vi "PS Control (OLD).vi"() -> ()   [LabVIEW 2013]
uses:
  <vilib>/rvi/interface/nirviOpenFPGA/nirviOpenFPGA.xnode
  <vilib>/rvi/interface/nirviReadWriteControl/nirviReadWriteControl.xnode
  <vilib>/rvi/interface/Simulation/niFpgaSimulationCallBeginRW.vi
  <vilib>/rvi/errors/niLvFpgaAdjustHostInterfaceError.vi
  <vilib>/addons/control/pid/NI_PID_pid.lvlib
  <vilib>/addons/control/pid/pid.llb/PID (DBL).vi
  <vilib>/ptbypt/NI_PtbyPt.lvlib
  <vilib>/Analysis/3filter.llb/Filter Passband Type.ctl
  <vilib>/Analysis/NI_AALBase.lvlib
  NiFpgaLv.dll
  <vilib>/Utility/error.llb/Error Cluster From Error Code.vi
  <vilib>/NI_Real-Time Target Support.lvlib
  FPGA Bitfiles/TIsbRIO_FPGATarget_pscontroldebug(f_tRBWsiwFJX4.lvbitx
  debug/ps control debug (fpga).vi
  <vilib>/FPGAPlugInAG/sbRIO-9626/niLvFpga_Open_sbRIO-9626.vi
  <vilib>/rvi/interface/common/dynamic/niFpgaDynamicAddResources.vi
panel:
  in  "feedforward":dbl
  out "Total (%)":dbl
  in  "Scale 2":dbl=2.0
  in  "Offset 2":dbl
  out "PS Feedback 2":dbl=1.3965510190723505
  in  "PS Cmd 2":dbl=13.5 format="%.2f"
  in  "PID gains 2":T1={"proportional gain (Kc)"=1.0, "integral time (Ti, min)"=0.01, "derivative time (Td, min)"=0.0} {"derivative time (Td, min)" format="%.3f"; "integral time (Ti, min)" format="%.3f"; "proportional gain (Kc)" format="%.3f"}
  in  "dt (s) 2":dbl=-1.0 format="%.3f"
  in  "output range 2":cluster{"output high":dbl, "output low":dbl}={"output high"=8.0, "output low"=0.0} {"output low" format="%.2f"; "output high" format="%.2f"}
  out "AO1":fxp<+/-,20,5>=0.7481689453125
  out "AI7":fxp<+/-,24,5>=0.5325374603271484
  out "AI6":fxp<+/-,24,5>=0.5325374603271484
  out "AO0":fxp<+/-,20,5>=0.7481689453125
  in  "output range":cluster{"output high":dbl, "output low":dbl}={"output high"=8.0, "output low"=0.0} {"output low" format="%.2f"; "output high" format="%.2f"}
  in  "dt (s)":dbl=-1.0 format="%.3f"
  in  "PID gains":T1={"proportional gain (Kc)"=1.0, "integral time (Ti, min)"=0.01, "derivative time (Td, min)"=0.0} {"derivative time (Td, min)" format="%.3f"; "integral time (Ti, min)" format="%.3f"; "proportional gain (Kc)" format="%.3f"}
  in  "PS Cmd 1":dbl=13.5 format="%.2f"
  out "PS Feedback 1":dbl=1.3965510190723505
  in  "Offset":dbl
  in  "Scale":dbl=2.0
  in  "Loop Timer (uSec)":u32=10000
  # "PS 1"
  # "PS 2"
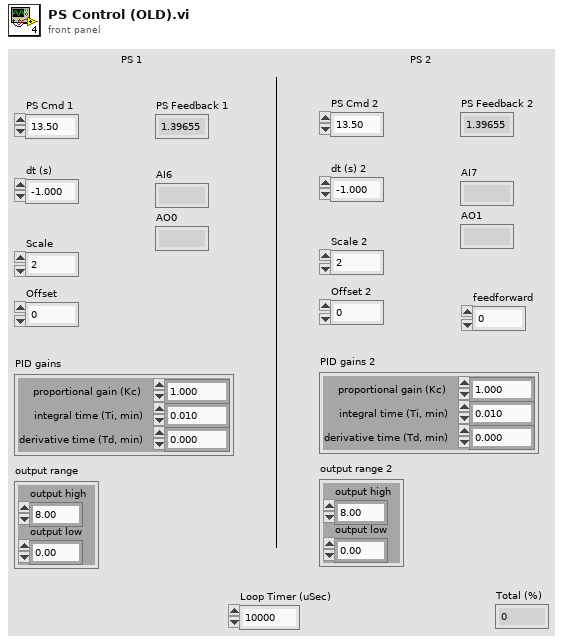
[diagram p1: front panel]
types:
  T1 = cluster{"proportional gain (Kc)":dbl, "integral time (Ti, min)":dbl, "derivative time (Td, min)":dbl}
  T2 = typedef "NI_AALBase.lvlib/Filter Passband Type.ctl" = enum32{"Lowpass", "Highpass", "Bandpass", "Bandstop"}
  T3 = typedef "NI_Real-Time Target Support.lvlib/RT CPU Load.ctl" = cluster{"Total (%)":dbl, "Time Critical (%)":dbl, "Timed Structures (%)":dbl, "High (%)":dbl, "Above Normal (%)":dbl, "Normal (%)":dbl, "Background (%)":dbl, "Idle (%)":dbl, "ISR (%)":dbl}
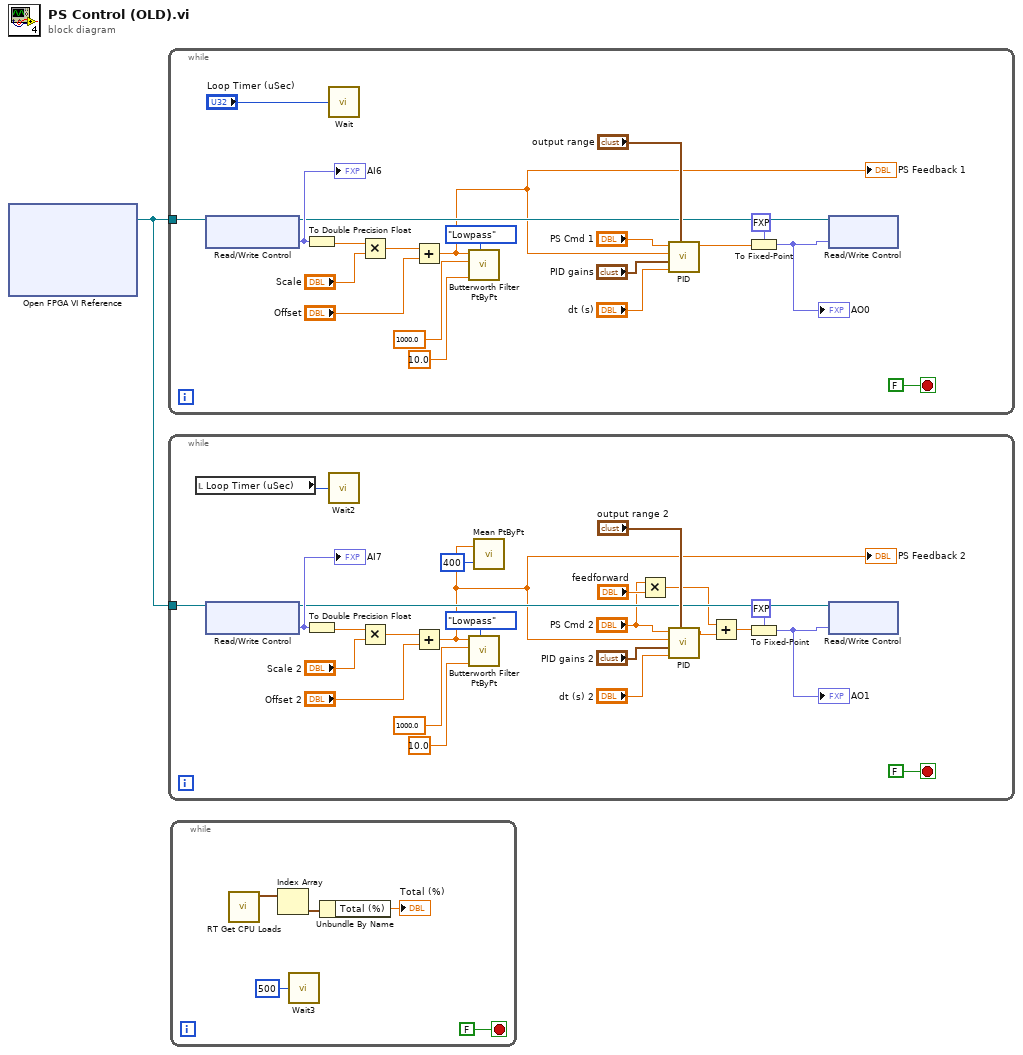
[diagram p0: block diagram]
diagram:
  n1 = xnode "Open FPGA VI Reference"() -> ("FPGA VI Reference Out"=w1:refnum<k20>)  [unwired: 2 in, 1 out]
  n2 = while {
    tunnel: w1 -> [w20]
    stop <- FALSE stop-if-true
    n3 = xnode "Read/Write Control"("FPGA VI Reference In"=w20) -> ("FPGA VI Reference Out"=w7:refnum<k20>, "PS Feedback 1"=w18:fxp<+/-,24,5>)  [unwired: 1 in, 1 out]
    "AI6" <- w18
    n4 = To Double Precision Float(number=w18) -> (double precision float=w6:dbl)
    n5 = call "Wait"("Count(uSec)"="Loop Timer (uSec)") -> ()  [unwired: 1 out]
    n6 = Multiply(x=w6, y="Scale") -> (x*y=w16:dbl)
    n7 = Add(x=w16, y="Offset") -> (x+y=w2:dbl)
    "PS Feedback 1" <- w2
    n8 = call <vilib>:"Butterworth Filter PtByPt.vi"("filter type"=Filter_Passband_Type."Lowpass", "low cutoff freq: fl"=10.0, "sampling freq: fs"=1000.0, "x"=w2) -> ()  [unwired: 5 in, 2 out]
    n9 = call-poly <vilib>:"PID.vi"("output range"="output range", "dt (s)"="dt (s)", "PID gains"="PID gains", "process variable"=w2, "setpoint"="PS Cmd 1") -> ("output"=w10:dbl)  [unwired: 5 in, 1 out]
    n10 = To Fixed-Point(fixed-point type=fxp<+/-,20,5> 0.0 ("PS Cmd"), number=w10) -> (fixed-point=w9:fxp<+/-,20,5>)
    "AO0" <- w9
    n11 = xnode "Read/Write Control"("FPGA VI Reference In"=w7, "PS Cmd 1"=w9) -> ()  [unwired: 1 in, 2 out]
  }
  n12 = while {
    tunnel: w1 -> [w44]
    stop <- FALSE stop-if-true
    n13 = local read "Loop Timer (uSec)"() -> (w29:u32)
    n14 = xnode "Read/Write Control"("FPGA VI Reference In"=w44) -> ("FPGA VI Reference Out"=w34:refnum<k20>, "PS Feedback 2"=w43:fxp<+/-,24,5>)  [unwired: 1 in, 1 out]
    "AI7" <- w43
    n15 = To Double Precision Float(number=w43) -> (double precision float=w33:dbl)
    n16 = call "Wait2"("Count(uSec)"=w29) -> ()  [unwired: 1 out]
    n17 = Multiply(x=w33, y="Scale 2") -> (x*y=w41:dbl)
    n18 = Add(x=w41, y="Offset 2") -> (x+y=w25:dbl)
    "PS Feedback 2" <- w25
    n19 = call <vilib>:"Butterworth Filter PtByPt.vi"("filter type"=Filter_Passband_Type."Lowpass", "low cutoff freq: fl"=10.0, "sampling freq: fs"=1000.0, "x"=w25) -> ()  [unwired: 5 in, 2 out]
    n20 = call <vilib>:"Mean PtByPt.vi"("x"=w25, "sample length"=400) -> ()  [unwired: 2 in, 2 out]
    n21 = Multiply(x="PS Cmd 2", y="feedforward") -> (x*y=w24:dbl)
    n22 = call-poly <vilib>:"PID.vi"("output range"="output range 2", "dt (s)"="dt (s) 2", "PID gains"="PID gains 2", "process variable"=w25, "setpoint"="PS Cmd 2") -> ("output"=w27:dbl)  [unwired: 5 in, 1 out]
    n23 = Add(x=w24, y=w27) -> (x+y=w26:dbl)
    n24 = To Fixed-Point(fixed-point type=fxp<+/-,20,5> 0.0 ("PS Cmd"), number=w26) -> (fixed-point=w36:fxp<+/-,20,5>)
    "AO1" <- w36
    n25 = xnode "Read/Write Control"("FPGA VI Reference In"=w34, "PS Cmd 2"=w36) -> ()  [unwired: 1 in, 2 out]
  }
  n26 = while {
    stop <- FALSE stop-if-true
    n27 = call <vilib>:"RT Get CPU Loads.vi"() -> ("CPU loads"=w50:T3[])  [unwired: 10 in, 1 out]
    n28 = Index Array(array=w50) -> (element=w49:T3)  [unwired: 1 in]
    n29 = call "Wait3"("Count(mSec)"=u32 500) -> ()  [unwired: 1 out]
    n30 = Unbundle By Name(w49) -> ("Total (%)"=→"Total (%)":dbl)
  }
